vi "RetrieveMeasurementMetadata.vi"(8 "error in (no error)":errorcluster, 11 "DatabaseConnectionInfo":T1) -> (0 "error out":errorcluster, 3 "MeasurementMetadata":string[][](array[string]))   [LabVIEW 2017]
uses:
  <vilib>/addons/database/Connection.llb/DB Tools Open Connec (Path).vi
  <vilib>/addons/database/_DB Variant To Data/Database Variant To Data.xnode
  <vilib>/addons/database/NI_Database_API.lvlib
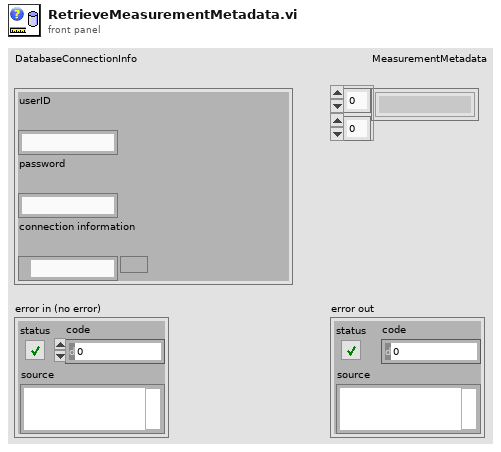
[diagram p1: front panel]
types:
  T1 = cluster{"userID":string, "password":string, "connection information":path}
  T2 = typedef "NI_Database_API.lvlib/Conn ObjectReference.ctl" = refnum<k1>
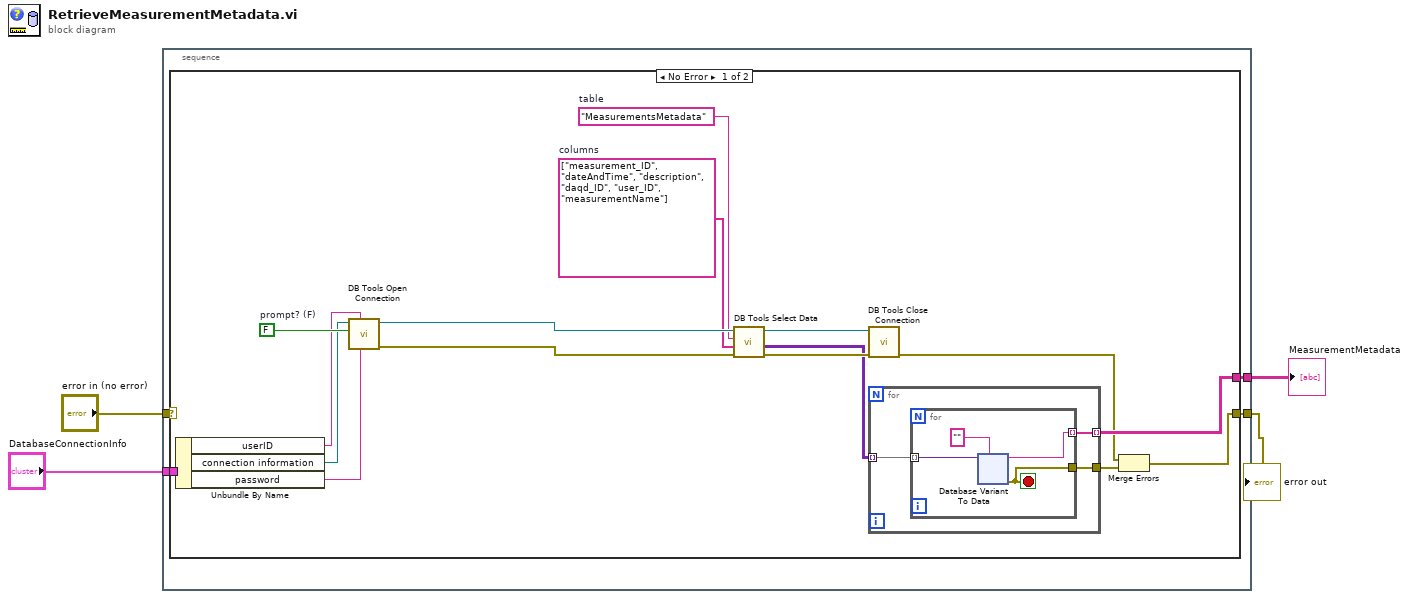
[diagram p0: block diagram]
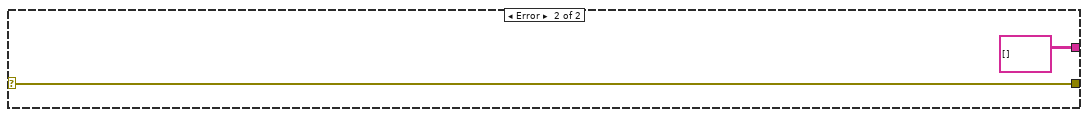
[diagram p2: hidden frame]
diagram:
  n1 = stacked-sequence {
    tunnel: [w8] -> w4
    tunnel: [w5] -> w3
    tunnel: "error in (no error)" -> [w7]
    tunnel: "DatabaseConnectionInfo" -> [w6]
    frame #0 {
      n2 = case shown="No Error" w7 {
        selector: w7 -> [_ w65]
        tunnel: [w24 string[][] []] -> w5
        tunnel: w6 -> [w23 _]
        tunnel: [w22 w65] -> w8
        frame No Error {
          w15 = string[] ["measurement_ID", "dateAndTime", "description", "daqd_ID", "user_ID", "measurementName"]  # columns
          w16 = "MeasurementsMetadata"  # table
          w21 = FALSE  # prompt? (F)
          n3 = Unbundle By Name(w23) -> ("userID"=w11:string, "connection information"=w9:path, "password"=w10:string)
          n4 = call-poly <vilib>:"DB Tools Open Connection.vi"("password"=w10, "userID"=w11, "prompt? (F)"=w21, "connection information"=w9) -> ("error out"=w19:errorcluster, "connection reference"=w18:T2)  [unwired: 4 in]
          n5 = call <vilib>:"DB Tools Select Data.vi"("error in (no error)"=w19, "columns"=w15, "table"=w16, "connection reference"=w18) -> ("error out"=w17:errorcluster, "data"=w14:variant[][], "connection reference out"=w20:T2)  [unwired: 2 in]
          n6 = call <vilib>:"DB Tools Close Connection.vi"("error in (no error)"=w17, "connection reference"=w20) -> ("error out"=w13:errorcluster)  [unwired: 5 in]
          n7 = for {
            tunnel: w14 -> [w27] mode=indexing
            tunnel: [w26] -> w12
            tunnel: [w25] -> w24 mode=indexing
            n8 = for {
              tunnel: w27 -> [w31] mode=indexing
              tunnel: [w29] -> w26
              tunnel: [w28] -> w25 mode=indexing
              stop <- w29 stop-if-true
              n9 = xnode "Database Variant To Data"("database variant"=w31, "type"="") -> ("data"=w28:string, "error out"=w29:errorcluster)  [unwired: 1 in]
            }
          }
          n10 = Merge Errors(w13, w12) -> (w22:errorcluster)
        }
        frame Error {
        }
      }
    }
  }
  "error out" <- w4
  "MeasurementMetadata" <- w3
